vi "SetImageBuffer.vi"(8 "error in (no error)":errorcluster, 9 "Image Type":T1=1 items=["Grayscale (U8)", "Grayscale (I16)", "Grayscale (SGL)", "Complex (CSG)", "RGB (U32)", "HSL (U32)", "RGB (U64)", "Grayscale (U16)"], 10 "max queue size (-1, unlimited)":i32, 11 "Camera_Prime95B in":refnum<class "Camera_Prime95B.lvclass">) -> (0 "error out":errorcluster, 3 "Camera_Prime95B out":refnum<class "Camera_Prime95B.lvclass">)   [LabVIEW 2020, in "Camera_Prime95B.lvlib" / "Camera_Prime95B.lvclass"]
uses:
  Camera_Prime95B.lvclass
  Camera_Prime95B.lvclass/Camera_Prime95B.ctl
  E:/Development/DevHardSoftware/MicroscopyFramework/Model/Hardware Layer/Real Hardware/Camera_Prime95B/Camera_Prime95B/Dependencies/PVCamNET.dll
  Dependencies/PVCamNET.dll
  Hardware Abstraction Layer/Component/Camera/Camera/Camera.lvclass
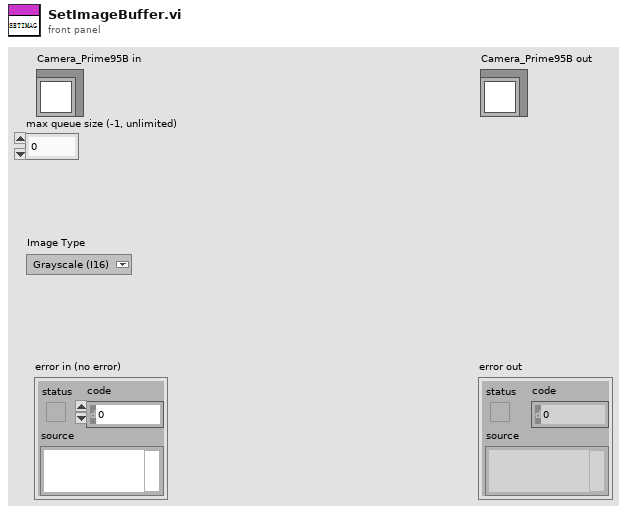
[diagram p1: front panel]
types:
  T1 = typedef "Image Type" = u32
  T2 = typedef "Device.lvlib/DeviceStatus.ctl" = i32
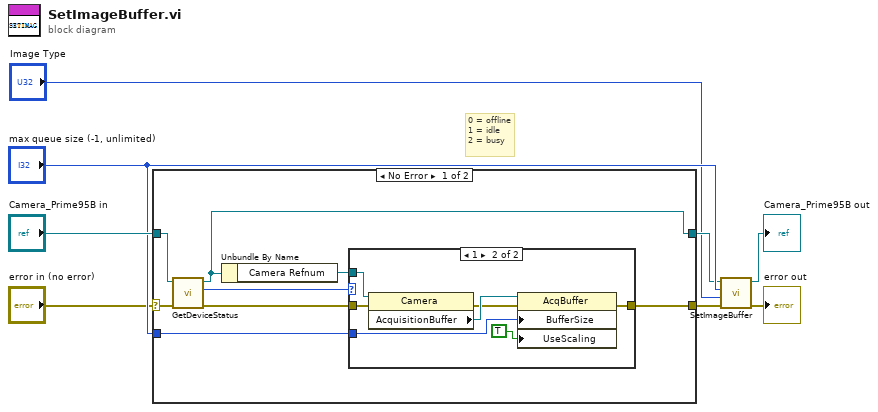
[diagram p0: block diagram]
diagram:
  # "0 = offline\n1 = idle\n2 = busy"
  n1 = case shown="No Error" "error in (no error)" {
    selector: "error in (no error)" -> [w14 w26]
    tunnel: [w15 w26] -> w4
    tunnel: "Camera_Prime95B in" -> [w13 w25]
    tunnel: "max queue size (-1, unlimited)" -> [w16 _]
    tunnel: [w9 w25] -> w3
    frame No Error {
      n2 = call-dynamic "GetDeviceStatus.vi"("error in (no error)"=w14, "Camera_Prime95B in"=w13) -> ("error out"=w12:errorcluster, "Status"=w10:T2, "Camera_Prime95B out"=w9:refnum<class "Camera_Prime95B.lvclass">)  [unwired: 7 in]
      n3 = Unbundle By Name(w9) -> ("Camera Refnum"=w11:refnum<k24>)
      n4 = case shown="1" w10 {
        tunnel: [w17 w24] -> w15
        tunnel: w16 -> [_ w21]
        tunnel: w12 -> [w17 w19]
        tunnel: w11 -> [_ w18]
        frame 0, Default {
        }
        frame 1 {
          n5 = property class="Camera"(reference=w18, error in=w19) -> (error out=w22:errorcluster, "AcquisitionBuffer"=w23:refnum<k24>)  [unwired: 1 out]
          n6 = property class="AcqBuffer"(reference=w23, error in=w22, "BufferSize"=w21, "UseScaling"=TRUE) -> (error out=w24:errorcluster)  [unwired: 1 out]
        }
      }
    }
    frame Error {
    }
  }
  n7 = call-parent "SetImageBuffer.vi"("error in (no error)"=w4, "Image Type"="Image Type", "BufferSize"="max queue size (-1, unlimited)", "Camera in"=w3) -> ("error out"=→"error out":errorcluster, "Camera out"=→"Camera_Prime95B out":refnum<class "Camera_Prime95B.lvclass">)  [unwired: 6 in]
